vi "Read All Washers.vi"(0 "Com Array":u8[](array[numeric]), 5 "HCC  Array In":T1[](array[typedef]), 7 "Partial Message Array":cluster{"Partial Message Out":u8[]}[](array[cluster]), 11 "error in (no error)":errorcluster) -> (4 "Log Coms Array":string[](array[string]), 6 "HCC  Array Out":T1[](array[typedef]), 8 "Data Present":bool[](array[boolean]), 10 "Partial Messages Out":cluster{"Partial Message Out":u8[]}[](array[cluster]), 15 "error out":errorcluster)   [LabVIEW 2011]
uses:
  HCC Data.ctl
  Washer Status Ctrl.ctl
  Globals HCC.vi
panel:
  out "Array":errorcluster[](array[cluster])
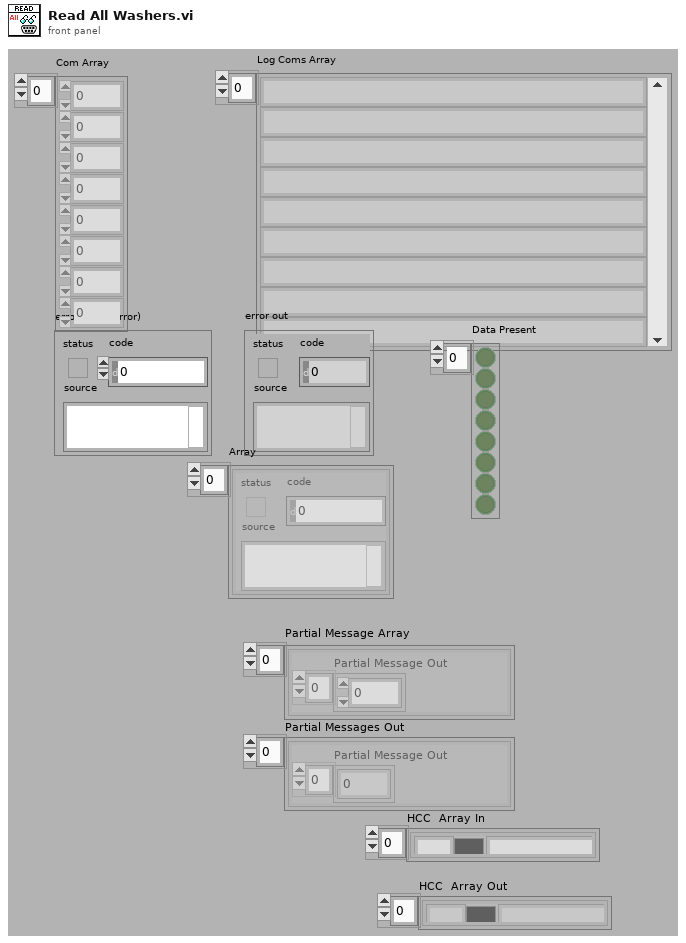
[diagram p1: front panel]
types:
  T1 = typedef "HCC Data.ctl" = cluster{"Station":string, "Color":u32, "Status":T2, "Error Time":string, "Com Err Count":u32, "Debug Log":string}
  T2 = typedef "Washer Status Ctrl.ctl" = enum16{"Running", "Err", "No Com", "No Conf"}
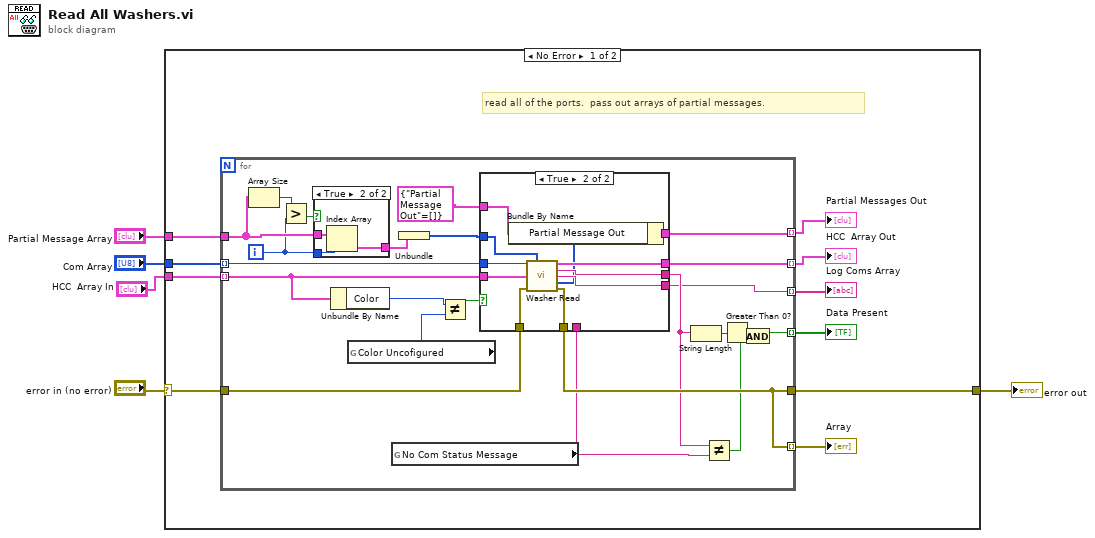
[diagram p0: block diagram]
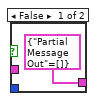
[diagram p2: hidden frame]
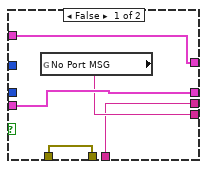
[diagram p3: hidden frame]
diagram:
  n1 = case shown="No Error" "error in (no error)" {
    selector: "error in (no error)" -> [w13 w58]
    tunnel: "Com Array" -> [w15 _]
    tunnel: [w12 w58] -> w4
    tunnel: "HCC  Array In" -> [w11 _]
    tunnel: "Partial Message Array" -> [w7 _]
    frame No Error {
      # "read all of the ports.  pass out arrays of partial messages."
      n2 = for {
        tunnel: w15 -> [w38] mode=indexing
        tunnel: w13 -> [w37]
        tunnel: [w35] -> w12
        tunnel: [w36] -> w6 mode=indexing
        tunnel: [w16] -> w14 mode=indexing
        tunnel: w11 -> [w29] mode=indexing
        tunnel: [w35] -> w9 mode=indexing
        tunnel: [w31] -> w8 mode=indexing
        tunnel: [w25] -> w10 mode=indexing
        tunnel: w7 -> [w21]
        i -> [w18]
        n3 = Array Size(array=w21) -> (size(s)=w19:i32)
        n4 = Greater?(x=w19, y=w18) -> (0:w20:bool)
        n5 = case shown="True" w20 {
          tunnel: [cluster{"Partial Message Out":u8[]} {"Partial Message Out"=[]} ("Cluster") w42] -> w22
          tunnel: w18 -> [_ w41]
          tunnel: w21 -> [_ w40]
          frame False {
          }
          frame True {
            n6 = Index Array(array=w40, index=w41) -> (element=w42:cluster{"Partial Message Out":u8[]})
          }
        }
        n7 = Unbundle By Name(w29) -> ("Color"=w27:u32)
        n8 = global read "Globals HCC.vi" "Color Uncofigured"() -> (w26:u32)
        n9 = global read "Globals HCC.vi" "No Com Status Message"() -> (w17:string)
        n10 = Unbundle(w22) -> ("Partial Message Out"=w23:u8[])
        n11 = Not Equal?(x=w27, y=w26) -> (x != y?=w28:bool)
        n12 = case shown="True" w28 {
          tunnel: w38 -> [_ w57]
          tunnel: w37 -> [w46 w56]
          tunnel: [w47 w55] -> w36
          tunnel: w29 -> [w47 w54]
          tunnel: [w46 w53] -> w35
          tunnel: [w45 w52] -> w16
          tunnel: [w44 w51] -> w32
          tunnel: w17 -> [w44 _]
          tunnel: [w43 w49] -> w25
          tunnel: cluster{"Partial Message Out":u8[]} {"Partial Message Out"=[]} ("Cluster") -> [w43 w49]
          tunnel: w23 -> [_ w48]
          frame False {
            n13 = global read "Globals HCC.vi" "No Port MSG"() -> (w45:string)
          }
          frame True {
            n14 = call "Washer Read.vi"("Com Chan"=w57, "Partial Message Start"=w48, "Washer Data In"=w54, "error in (no error)"=w56) -> ("Washer Data Out"=w55:T1, "Read Buffer"=w51:string, "Log String"=w52:string, "Partial Message Out"=w50:u8[], "error out"=w53:errorcluster)  [unwired: 7 in]
            n15 = Bundle By Name(cluster=w49, "Partial Message Out"=w50) -> ()  [unwired: 1 out]
          }
        }
        n16 = String Length(string=w32) -> (length=w34:i32)
        n17 = Not Equal?(x=w32, y=w17) -> (x != y?=w30:bool)
        n18 = Greater Than 0?(x=w34) -> (x > 0?=w33:bool)
        n19 = And(x=w33, y=w30) -> (x .and. y?=w31:bool)
      }
      "Log Coms Array" <- w14
      "Partial Messages Out" <- w10
      "Array" <- w9
      "Data Present" <- w8
      "HCC  Array Out" <- w6
    }
    frame Error {
    }
  }
  "error out" <- w4
